vi "clear Session Data.vi"(0 "Session in":refnum<class "SequenceFile.lvclass">, 11 "error in":errorcluster) -> (4 "Session out":refnum<class "SequenceFile.lvclass">, 15 "error out":errorcluster)   [LabVIEW 2020, in "HTS.lvlib" / "SequenceFile.lvclass"]
uses:
  SequenceFile.lvclass
  SequenceFile.lvclass/SequenceFile.ctl
  <userlib>/_Session Fwk/Session - Root.lvclass
  Engine/Engine.lvclass
  VariableContainer/VariableContainer.lvclass
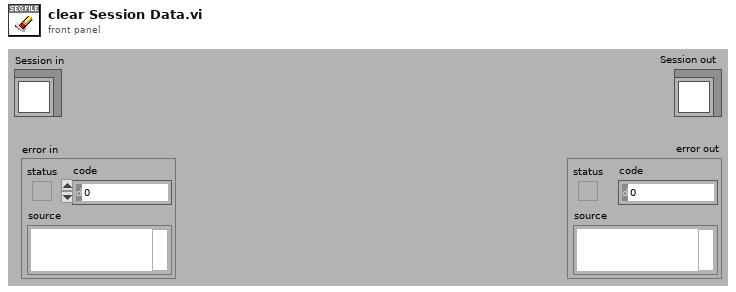
[diagram p1: front panel]
types:
  T1 = typedef "HTS.lvlib/Engine.lvclass/Session Handle.ctl" = refnum<data-value>
  T2 = typedef "HTS.lvlib/VariableContainer.lvclass/Session Handle.ctl" = refnum<data-value>
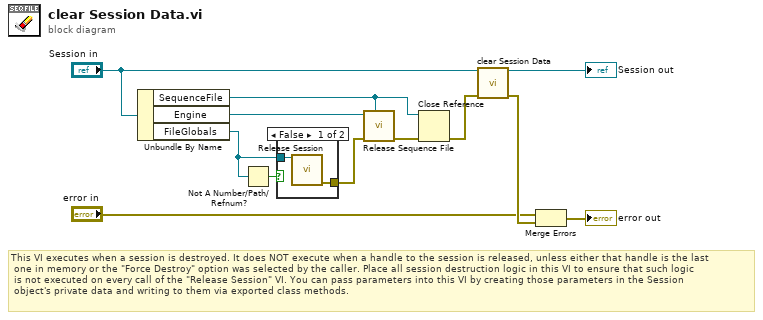
[diagram p0: block diagram]
diagram:
  # "This VI executes when a session is destroyed. It does NOT execute when a handle to the session is released, unless either that handle is the last\n one in memory or the \"Force Destroy\" option was selected by the caller. Place all session destruction logic in this VI to ensure that such logic\n is not executed on every call of the \"Release Session\" VI. You can pass parameters into this VI by creating those parameters in the Session \n object's private data and writing to them via exported class methods."
  n1 = Unbundle By Name("Session in") -> ("SequenceFile"=w7:refnum<k7>, "Engine"=w9:T1, "FileGlobals"=w2:T2)
  n2 = Not A Number/Path/Refnum?(number/path/refnum=w2) -> (NaN/Path/Refnum?=w1:bool)
  n3 = case shown="False" w1 {
    tunnel: w2 -> [w14 _]
    tunnel: [w13 _] -> w3
    frame False {
      n4 = call "Release Session.vi"("Session Handle"=w14) -> ("error out"=w13:errorcluster)  [unwired: 14 in]
    }
    frame True {
    }
  }
  n5 = call "Release Sequence File.vi"("SequenceFile"=w7, "error in (no error)"=w3, "Session Handle in"=w9) -> ("error out"=w8:errorcluster)  [unwired: 7 in, 1 out]
  n6 = Close Reference(reference=w7, error in (no error)=w8) -> (error out=w6:errorcluster)
  n7 = call-parent "clear Session Data.vi"("OBJ - Measurement Session in"="Session in", "error in"=w6) -> ("OBJ - Measurement Session out"=→"Session out":refnum<class "SequenceFile.lvclass">, "error out"=w11:errorcluster)  [unwired: 12 in]
  n8 = Merge Errors("error in", w11) -> (→"error out":errorcluster)
